vi "Transfer_Chunk_U16_IMG_to_Str_2.vi"(2 "error IN":errorcluster, 3 "[IN] Use remained rows":bool, 4 "[IN] # rows last transfer":i32, 5 "[IN] # rows single transfer":i32, 6 "[IN] # of chunk":i32, 7 "[IN] U16 Pixel Img":u16[][](array[numeric])) -> (0 "error OUT":errorcluster, 1 "[OUT] Converted String":string)   [LabVIEW 2020]
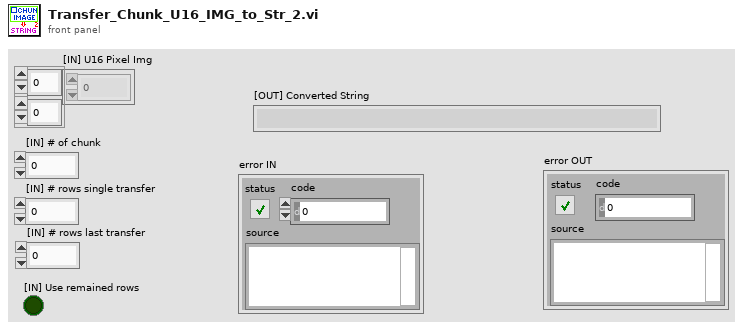
[diagram p1: front panel]
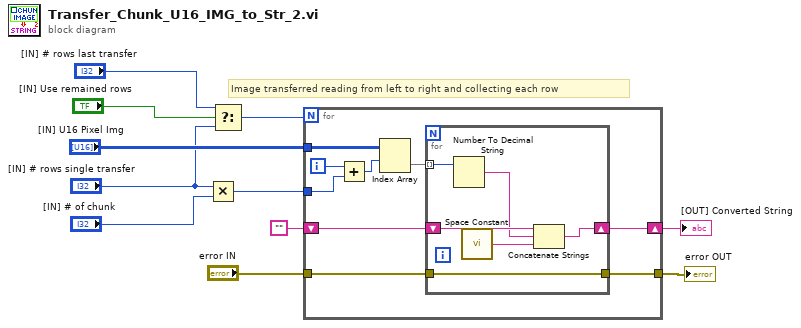
[diagram p0: block diagram]
diagram:
  # "Image transferred reading from left to right and collecting each row"
  n1 = Multiply(x="[IN] # rows single transfer", y="[IN] # of chunk") -> (x*y=w7:i32)
  n2 = Select(t="[IN] # rows last transfer", s="[IN] Use remained rows", f="[IN] # rows single transfer") -> (s? t:f=w4:i32)
  n3 = for {
    N: w4 -> [_]
    tunnel: "[IN] U16 Pixel Img" -> [w20]
    shift-right: [w18] -> w9
    shift-left: "" -> [w19]
    tunnel: w7 -> [w15]
    tunnel: "error IN" -> [w13]
    tunnel: [w12] -> w1
    i -> [w16]
    n4 = Add(x=w16, y=w15) -> (x+y=w14:i32)
    n5 = Index Array(array=w20, index (row)=w14) -> (element=w17:u16[])  [unwired: 1 in]
    n6 = for {
      tunnel: w17 -> [w26] mode=indexing
      shift-right: [w22] -> w18
      shift-left: w19 -> [w25]
      tunnel: w13 -> [w21]
      tunnel: [w21] -> w12
      n7 = Number To Decimal String(number=w26) -> (decimal integer string=w24:string)  [unwired: 1 in]
      n8 = call <vilib>:"Space Constant.vi"() -> ("String"=w23:string)
      n9 = Concatenate Strings(w25, w24, w23) -> (w22:string)
    }
  }
  "[OUT] Converted String" <- w9
  "error OUT" <- w1
